vi "svfa_Check for Frequency Range Change.vi"(6 "frequency range in":T1={"start frequency"=20.0, "stop frequency"=20000.0} {"stop frequency" format="%.2f"; "start frequency" format="%.2f"}, 7 "restart averaging (F)":bool, 8 "error in (no error)":errorcluster, 10 "dt":dbl) -> (0 "error out":errorcluster, 2 "Param_has_changed":bool, 4 "frequency range out":T1={"start frequency"=20.0, "stop frequency"=20000.0} {"stop frequency" format="%.2f"; "start frequency" format="%.2f"})   [LabVIEW 2017]
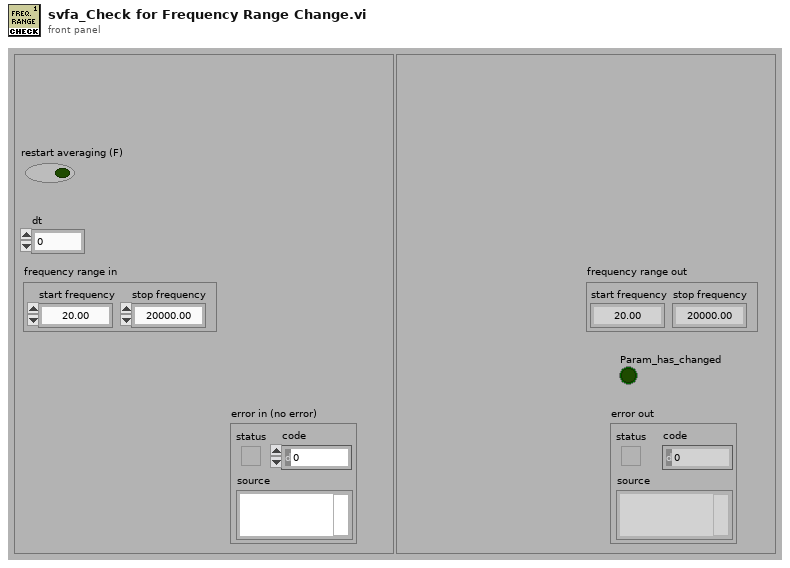
[diagram p1: front panel]
types:
  T1 = cluster{"start frequency":dbl, "stop frequency":dbl}
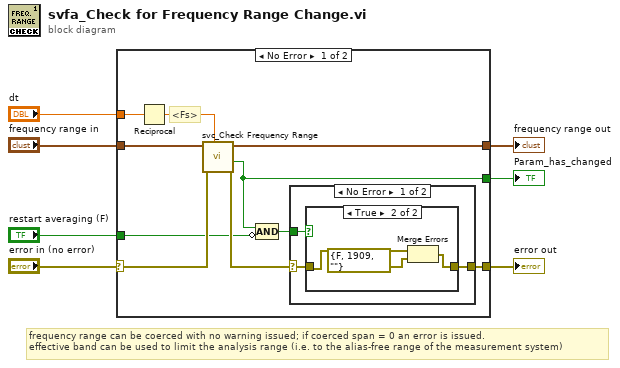
[diagram p0: block diagram]
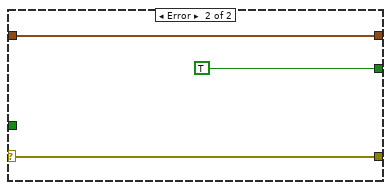
[diagram p4: hidden frame]
diagram:
  # "frequency range can be coerced with no warning issued; if coerced span = 0 an error is issued.\neffective band can be used to limit the analysis range (i.e. to the alias-free range of the measurement system)"
  n1 = case shown="No Error" "error in (no error)" {
    selector: "error in (no error)" -> [w16 w28]
    tunnel: "frequency range in" -> [w12 w26]
    tunnel: [w9 TRUE] -> w6
    tunnel: [w17 w28] -> w4
    tunnel: [w14 w26] -> w3
    tunnel: "dt" -> [w11 _]
    tunnel: "restart averaging (F)" -> [w10 _]
    frame No Error {
      # "<Fs>"
      n2 = Reciprocal(x=w11) -> (1/x=w13:dbl)
      n3 = call <vilib>:"svc_Check Frequency Range.vi"("fs"=w13, "error in (no error)"=w16, "frequency range in"=w12) -> ("error out"=w15:errorcluster, "frequency range changed"=w9:bool, "frequency range out"=w14:T1)  [unwired: 6 in]
      n4 = Compound Arithmetic op=AND(w9, invert w10) -> (w8:bool)
      n5 = case shown="No Error" w15 {
        selector: w15 -> [w18 w25]
        tunnel: w8 -> [w20 _]
        tunnel: [w19 w25] -> w17
        frame No Error {
          n6 = case shown="True" w20 {
            tunnel: w18 -> [w21 w24]
            tunnel: [w21 w22] -> w19
            frame False {
            }
            frame True {
              n7 = Merge Errors(w24, errorcluster {"status"=FALSE, "code"=1909, "source"=""} ("error IO")) -> (w22:errorcluster)
            }
          }
        }
        frame Error {
        }
      }
    }
    frame Error {
    }
  }
  "error out" <- w4
  "Param_has_changed" <- w6
  "frequency range out" <- w3
